vi "ReportTravelSpeed.vi"(1 "Speed":dbl=2.0, 2 "Destination":T1={"Subsystem Id"=90, "Node Id"=1, "Component Id"=1}, 3 "Source":T1={"Subsystem Id"=3, "Node Id"=1, "Component Id"=1}) -> (0 "Encoded JAUS Message":string)   [LabVIEW 2009]
uses:
  Support Files/Address.ctl
panel:
  in  "Command Code":string="D\n"
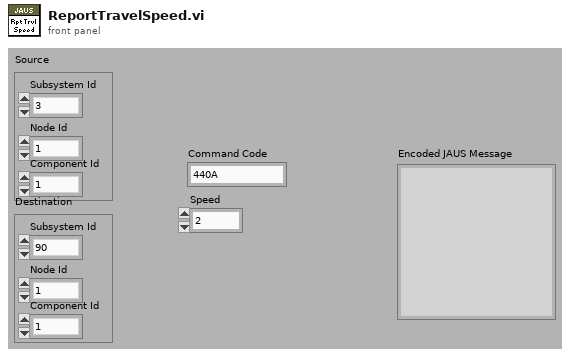
[diagram p1: front panel]
types:
  T1 = typedef "Address.ctl" = cluster{"Subsystem Id":u16, "Node Id":u8, "Component Id":u8}
  T2 = cluster{"unsigned byte array[0]":u8, "unsigned byte array[1]":u8}
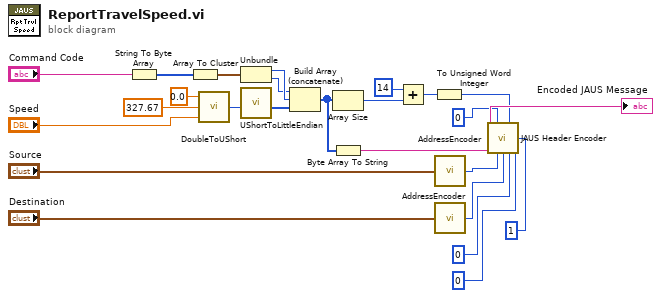
[diagram p0: block diagram]
diagram:
  n1 = String To Byte Array(string="Command Code") -> (unsigned byte array=w12:u8[])
  n2 = Array To Cluster(array=w12) -> (cluster=w11:T2)
  n3 = call "DoubleToUShort.vi"("Value"="Speed", "Max"=327.67, "Min"=0.0) -> ("scaled Integer"=w4:u16)
  n4 = Unbundle(w11) -> ("unsigned byte array[0]"=w10:u8, "unsigned byte array[1]"=w9:u8)
  n5 = call "UShortToLittleEndian.vi"("Number"=w4) -> ("byte array"=w3:u8[])  [unwired: 10 in]
  n6 = Build Array (concatenate)(w9, w10, w3) -> (w16:u8[])
  n7 = Array Size(array=w16) -> (size(s)=w14:i32)
  n8 = Byte Array To String(unsigned byte array=w16) -> (string=w18:string)
  n9 = Add(x=14, y=w14) -> (x+y=w13:i32)
  n10 = To Unsigned Word Integer(number=w13) -> (unsigned 16bit integer=w6:u16)
  n11 = call "AddressEncoder.vi"("Address Cluster"="Source") -> ("Address"=w24:u32)
  n12 = call "AddressEncoder.vi"("Address Cluster"="Destination") -> ("Address"=w23:u32)
  n13 = call "JAUS Header Encoder.vi"("Message Type (0-5)"=u8 0, "Data Size (8-23)"=w6, "Priority(40-41)"=u8 1, "Payload"=w18, "Source ID (80-95)"=w24, "Destination ID (48-79)"=w23, "Data Flags (46-47)"=u8 0, "Ack/Nak (44-45)"=u8 0) -> ("Encoded JAUS Message"=→"Encoded JAUS Message":string)  [unwired: 7 in]
